vi "Write Spectrum Analyzer.lvclass.vi"(10 "Spectrum Analyzer.lvclass":refnum<class "Spectrum Analyzer.lvclass">, 11 "MCCW ACLR in":refnum<class "MCCW ACLR.lvclass">) -> (3 "MCCW ACLR out":refnum<class "MCCW ACLR.lvclass">)   [LabVIEW 2020, in "MCCW ACLR.lvclass"]
uses:
  MCCW ACLR.lvclass
  Instruments/Spectrum Analyzer/Spectrum Analyzer.lvclass
  MCCW ACLR.lvclass/MCCW ACLR.ctl
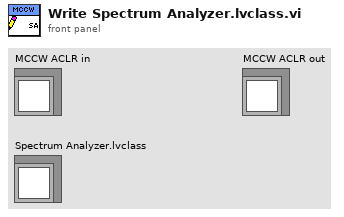
[diagram p1: front panel]
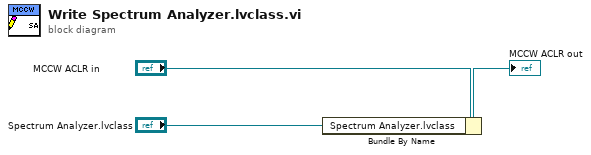
[diagram p0: block diagram]
diagram:
  n1 = Bundle By Name(cluster="MCCW ACLR in", "Spectrum Analyzer.lvclass"="Spectrum Analyzer.lvclass") -> (→"MCCW ACLR out":refnum<class "MCCW ACLR.lvclass">)
